vi "Sinus - Kopie.vi"(1 "Phi":dbl(slide) scale=0.0..3.14159, 2 "A":dbl(slide) scale=0.0..10.0, 3 "f":dbl(slide) scale=0.0..100.0, 4 "N":i32(slide) scale=0.0..1000.0) -> (0 "sin(x, t_i)":cluster{dbl[], dbl[]})   [LabVIEW 2017]
panel:
  out "XY Graph 2":cluster{dbl[], dbl[]}(graph)
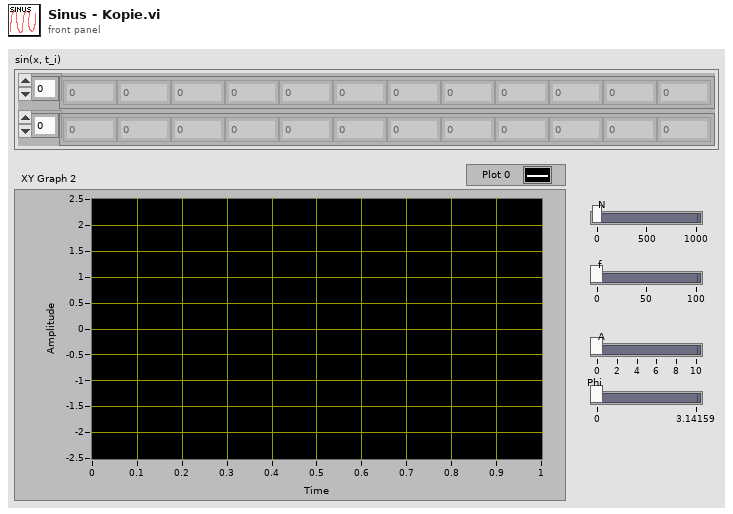
[diagram p1: front panel]
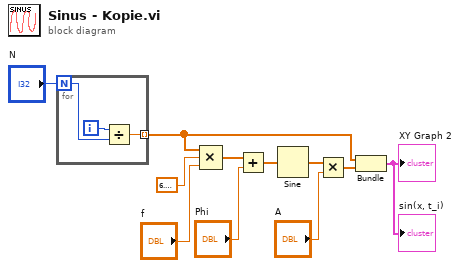
[diagram p0: block diagram]
diagram:
  n1 = for {
    N: "N" -> [w14]
    tunnel: [w12] -> w2 mode=indexing
    i -> [w13]
    n2 = Divide(x=w13, y=w14) -> (x/y=w12:dbl)
  }
  n3 = Compound Arithmetic op=MULTIPLY(w2, 6.283185307179586, "f") -> (w8:dbl[])
  n4 = Add(x=w8, y="Phi") -> (x+y=w6:dbl[])
  n5 = Sine(x=w6) -> (sin(x)=w5:dbl[])
  n6 = Multiply(x=w5, y="A") -> (x*y=w1:dbl[])
  n7 = Bundle(w2, w1) -> (→"XY Graph 2" →"sin(x, t_i)":cluster{dbl[], dbl[]})  [unwired: 1 in]
